vi "Volts_to_temperature_(SubVI).vi"(4 "ch_data_string":string, 6 "Boolean in":bool, 7 "error in":errorcluster, 17 "koeff. cluster":T1) -> (20 "T solvation":dbl, 21 "meas_voltage":dbl, 26 "Boolean out":bool, 27 "error out":errorcluster)   [LabVIEW 2015]
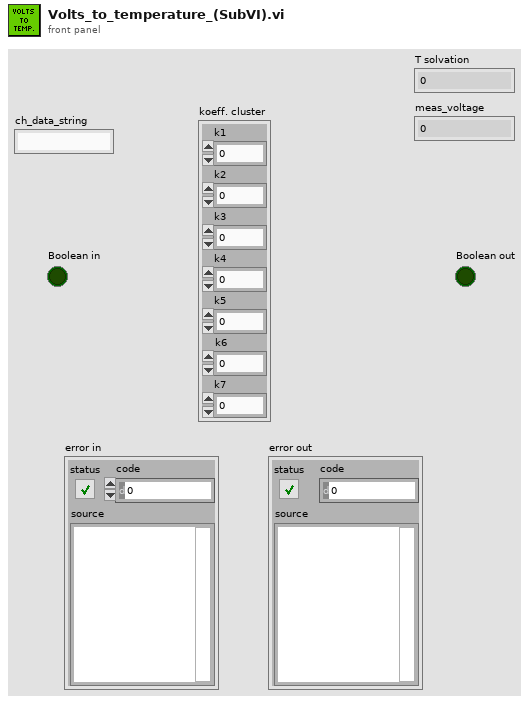
[diagram p1: front panel]
types:
  T1 = cluster{"k1":ext, "k2":ext, "k3":ext, "k4":ext, "k5":ext, "k6":ext, "k7":ext}
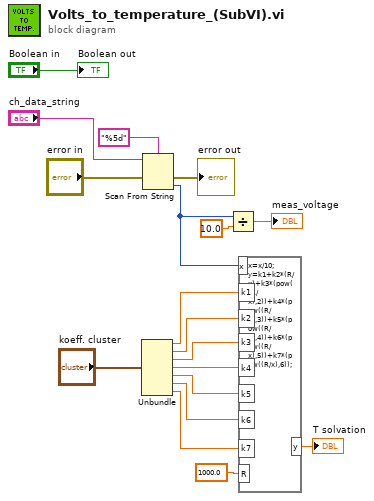
[diagram p0: block diagram]
diagram:
  n1 = Unbundle("koeff. cluster") -> ("k1"=w8:ext, "k2"=w7:ext, "k3"=w6:ext, "k4"=w5:ext, "k5"=w4:ext, "k6"=w3:ext, "k7"=w2:ext)
  n2 = Scan From String(format string="%5d", input string="ch_data_string", error in="error in") -> (error out=→"error out":errorcluster, output 1=w13:i32)  [unwired: 2 in, 2 out]
  n3 = Divide(x=w13, y=10.0) -> (x/y=→"meas_voltage":dbl)
  n4 = formula code="x=x/10;\ny=k1+k2*(R/x)+k3*(pow((R/x),2))+k4*(pow((R/x),3))+k5*(pow((R/x),4))+k6*(pow((R/x),5))+k7*(pow((R/x),6));"("x"=w13, "k1"=w8, "k2"=w7, "k3"=w6, "k4"=w5, "k5"=w4, "k6"=w3, "k7"=w2, "R"=1000.0 ("y")) -> ("y"=→"T solvation":dbl)
  "Boolean out" <- "Boolean in"
